vi "BLE_Read_Characteristic.vi"(0 ".NET Refnum in":refnum<k24>, 7 "CharacteristicUUID":string, 11 "error in (no error)":errorcluster) -> (4 ".NET Refnum out":refnum<k24>, 6 "ServicesUUIDs Value":string, 8 "number":u8[](array[numeric]), 10 "Engineering Value":string, 15 "error out":errorcluster)   [LabVIEW 2020, in "BLE.lvlib"]
uses:
  C:/Users/Trait/Desktop/LabView Project/LabView BLE DataACQ/BLELib.dll
  BLELib.dll
  BLE.lvlib
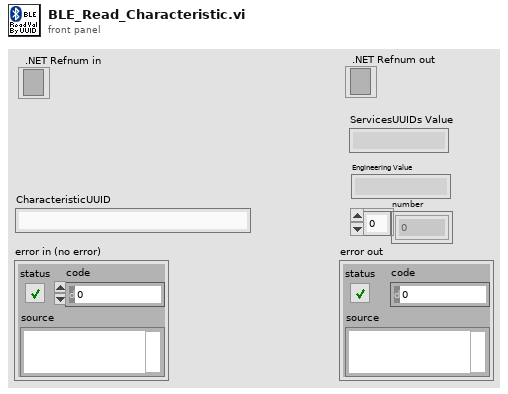
[diagram p1: front panel]
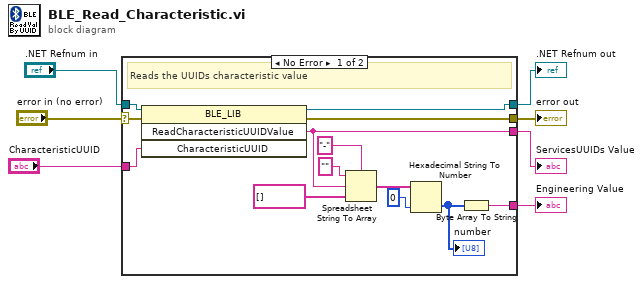
[diagram p0: block diagram]
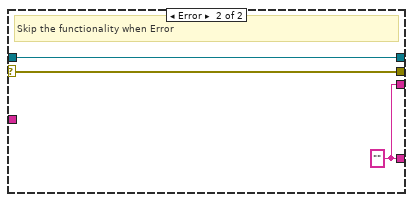
[diagram p2: hidden frame]
diagram:
  n1 = case shown="No Error" "error in (no error)" {
    selector: "error in (no error)" -> [w20 w22]
    tunnel: [w19 w23] -> w6
    tunnel: ".NET Refnum in" -> [w18 w23]
    tunnel: [w8 w22] -> w4
    tunnel: [w9 w21] -> w2
    tunnel: "CharacteristicUUID" -> [w12 _]
    tunnel: [w10 w21] -> w1
    frame No Error {
      # "Reads the UUIDs characteristic value"
      n2 = invoke class="BLE_LIB" method="ReadCharacteristicUUIDValue"(reference=w18, error in=w20, "CharacteristicUUID"=w12) -> (reference out=w19:refnum<k24>, error out=w8:errorcluster, "ReadCharacteristicUUIDValue"=w9:string)  [unwired: 1 in, 1 out]
      n3 = Spreadsheet String To Array(delimiter (Tab)="-", format string="", spreadsheet string=w9, array type (2D Dbl)=string[] []) -> (array=w14:string[])
      n4 = Hexadecimal String To Number(string=w14, default (0uL)=u8 0 ("default (0 U32)")) -> (number=w11:u8[])  [unwired: 1 in, 1 out]
      "number" <- w11
      n5 = Byte Array To String(unsigned byte array=w11) -> (string=w10:string)
    }
    frame Error {
      w21 = "" ("Result")
      # "Skip the functionality when Error"
    }
  }
  "error out" <- w4
  ".NET Refnum out" <- w6
  "ServicesUUIDs Value" <- w2
  "Engineering Value" <- w1
